vi "first test.vi"() -> ()   [LabVIEW 2022 SP3]
uses:
  <vilib>/Instr/_visa.llb/VISA Configure Serial Port (Instr).vi
panel:
  out "number":i32
  in  "stop":bool
  in  "baud rate (9600)":u32=9600
  in  "VISA resource name":refnum<visa-resource-name>
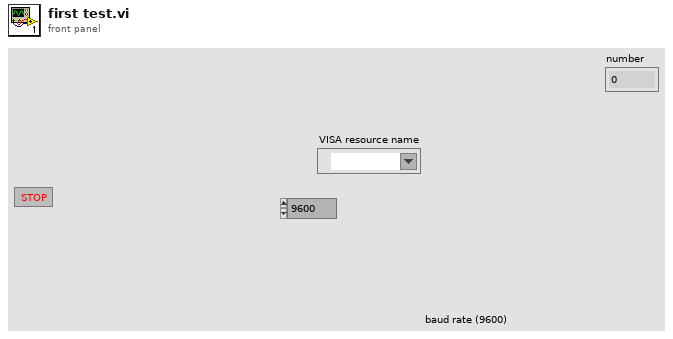
[diagram p1: front panel]
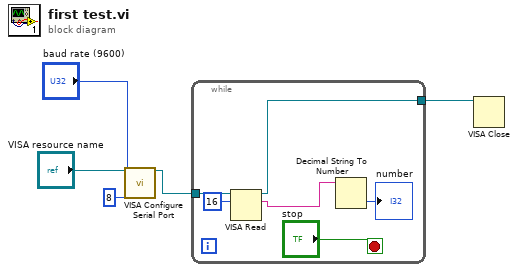
[diagram p0: block diagram]
diagram:
  n1 = call-poly "VISA Configure Serial Port"("VISA resource name"="VISA resource name", "baud rate (9600)"="baud rate (9600)", "data bits (8)"=u16 8) -> ("VISA resource name out"=w4:refnum<visa-resource-name>)  [unwired: 11 in, 1 out]
  n2 = while {
    tunnel: w4 -> [w11]
    tunnel: [w8] -> w1
    stop <- "stop" stop-if-true
    n3 = VISA Read(VISA resource name=w11, byte count=u32 16) -> (VISA resource name out=w8:refnum<visa-resource-name>, read buffer=w7:string)  [unwired: 1 in, 2 out]
    n4 = Decimal String To Number(string=w7) -> (number=→"number":i32)  [unwired: 2 in, 1 out]
  }
  n5 = VISA Close(VISA resource name=w1) -> ()  [unwired: 1 in, 1 out]
